vi "Error Refresh.vi"() -> (0 "Error Data":T1={"Motor Status"=TRUE, "LIDAR Status"=TRUE, "GPS Status"=TRUE, "LIDAR"={"status"=FALSE, "code"=0, "source"=""}, "GPS"={"status"=FALSE, "code"=0, "source"=""}, "Motor"={"status"=FALSE, "code"=0, "source"=""}})   [LabVIEW 2011]
panel:
  in  "Errors":T1={"Motor Status"=TRUE, "LIDAR Status"=TRUE, "GPS Status"=TRUE, "LIDAR"={"status"=FALSE, "code"=0, "source"=""}, "GPS"={"status"=FALSE, "code"=0, "source"=""}, "Motor"={"status"=FALSE, "code"=0, "source"=""}}
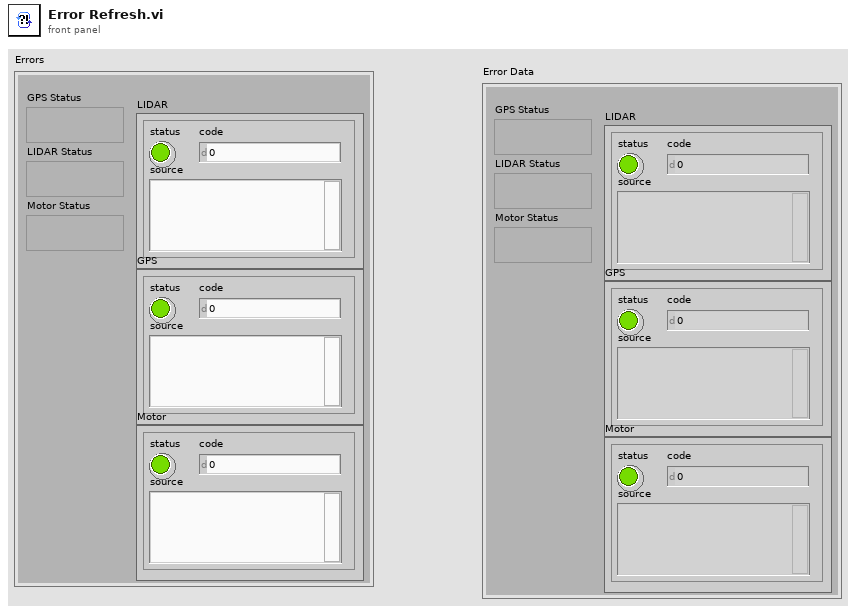
[diagram p1: front panel]
types:
  T1 = cluster{"Motor Status":bool, "LIDAR Status":bool, "GPS Status":bool, "LIDAR":errorcluster, "GPS":errorcluster, "Motor":errorcluster}
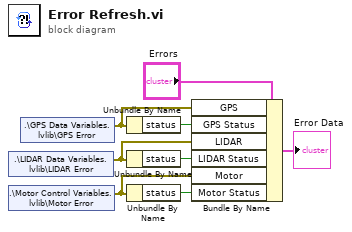
[diagram p0: block diagram]
diagram:
  n1 = shared-variable ".\\LIDAR Data Variables.lvlib\\LIDAR Error"() -> (w4:errorcluster)  [unwired: 1 in, 1 out]
  n2 = shared-variable ".\\Motor Control Variables.lvlib\\Motor Error"() -> (w2:errorcluster)  [unwired: 1 in, 1 out]
  n3 = shared-variable ".\\GPS Data Variables.lvlib\\GPS Error"() -> (w6:errorcluster)  [unwired: 1 in, 1 out]
  n4 = Unbundle By Name(w6) -> ("status"=w5:bool)
  n5 = Unbundle By Name(w4) -> ("status"=w3:bool)
  n6 = Unbundle By Name(w2) -> ("status"=w1:bool)
  n7 = Bundle By Name(cluster="Errors", "GPS"=w6, "GPS Status"=w5, "LIDAR"=w4, "LIDAR Status"=w3, "Motor"=w2, "Motor Status"=w1) -> (→"Error Data":T1)
